vi "BuildDAQCardChannelArray.vi"(11 "DAQ Channel Array":T1) -> (0 "Channel":tag[](array[tag]), 1 "Channel Name":string[](array[string]), 2 "Voltage Range":dbl[](array[numeric]), 3 "Active":bool[](array[boolean]))   [LabVIEW 2013]
uses:
  Controls/DAQ Card Channel Array.ctl
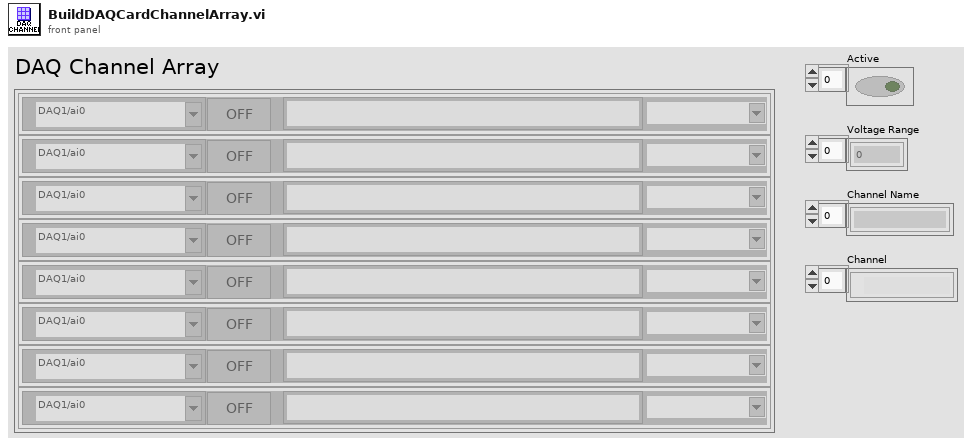
[diagram p1: front panel]
types:
  T1 = typedef "DAQ Card Channel Array.ctl" = cluster{"Active":bool, "Channel Name":string, "Channel":tag, "Voltage Range":string}[]
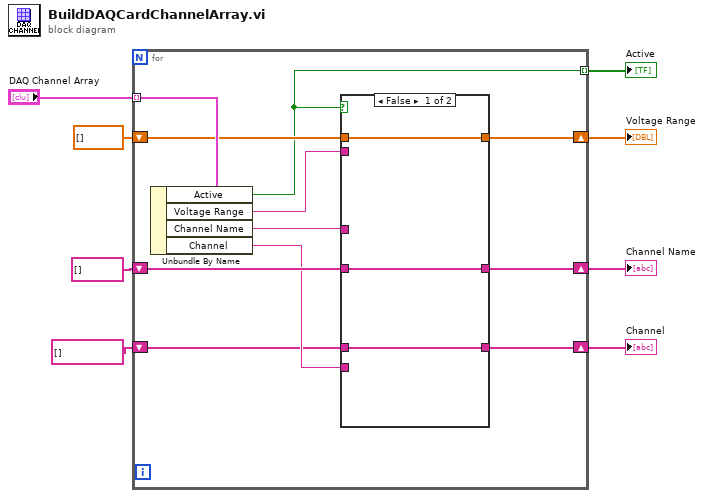
[diagram p0: block diagram]
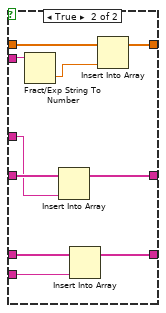
[diagram p2: hidden frame]
diagram:
  n1 = for {
    tunnel: "DAQ Channel Array" -> [w19] mode=indexing
    shift-right: [w18] -> w1
    shift-left: dbl[] [] -> [w17]
    shift-right: [w14] -> w3
    shift-left: string[] [] -> [w13]
    shift-right: [w11] -> w4
    shift-left: tag[] [] -> [w10]
    tunnel: [w9] -> w6 mode=indexing
    n2 = Unbundle By Name(w19) -> ("Active"=w9:bool, "Voltage Range"=w16:string, "Channel Name"=w15:string, "Channel"=w12:tag)
    n3 = case shown="False" w9 {
      tunnel: [w22 w32] -> w18
      tunnel: w17 -> [w22 w31]
      tunnel: w16 -> [_ w25]
      tunnel: w15 -> [_ w23]
      tunnel: [w21 w30] -> w14
      tunnel: w13 -> [w21 w29]
      tunnel: w12 -> [_ w28]
      tunnel: [w20 w27] -> w11
      tunnel: w10 -> [w20 w26]
      frame False {
      }
      frame True {
        n4 = Fract/Exp String To Number(string=w25) -> (number=w24:dbl)  [unwired: 3 in, 1 out]
        n5 = Insert Into Array(array=w29, new element=w23) -> (w30:string[])  [unwired: 1 in]
        n6 = Insert Into Array(array=w26, new element=w28) -> (w27:tag[])  [unwired: 1 in]
        n7 = Insert Into Array(array=w31, new element=w24) -> (w32:dbl[])  [unwired: 1 in]
      }
    }
  }
  "Active" <- w6
  "Channel" <- w4
  "Channel Name" <- w3
  "Voltage Range" <- w1
